vi "Autonomous Independent.vi"() -> ()   [LabVIEW 2013]
doc: "This VI is called when autonomous begins, and will automatically be terminated when autonomous ends. You can carry out timed or sensor driven robot movement independently without needing to return to the caller."
uses:
  <vilib>/Rock Robotics/WPI/SafetyOutput/WPI_SafetyOutputConfigMenu.ctl
  Robot Global Data.vi
  <vilib>/Rock Robotics/WPI/RobotDrive/WPI_RobotDriveGetSetRefNum.vi
  <vilib>/Rock Robotics/WPI/Joystick/WPI_JoystickGetSetRefNum.vi
  <vilib>/Rock Robotics/WPI/RobotDrive/WPI_RobotDriveArcadeDrive_Standard(NoSaturation).vi
panel:
  in  "Mantis_Arm_Move_Position":dbl=69.0
  in  "Max_Position_Error":dbl=5.0 format="%#_13g"
  in  "Shooting_Arm_Position":dbl=95.0
  in  "Min_Wait_Time":dbl=0.75
  in  "Right_Gain":dbl=0.95
  in  "Left_Gain":dbl=1.0
  in  "Backwards":bool
  in  "Invert_Right":bool=TRUE
  in  "Invert_Left":bool=TRUE
  out "Drive_Time_Actual":dbl=4.669
  in  "Loop_Rate":dbl=0.01
  in  "Ramp_Down_Time":dbl=1.0000000000000002
  in  "Hold_Time":dbl=2.85
  in  "Max_Speed":dbl=0.19999999999999968
  in  "Ramp_Up_Time":dbl=0.75
  # "Be sure to right-click and choose Data Operations>>Make Current Value default if you want to save the array values with the VI"
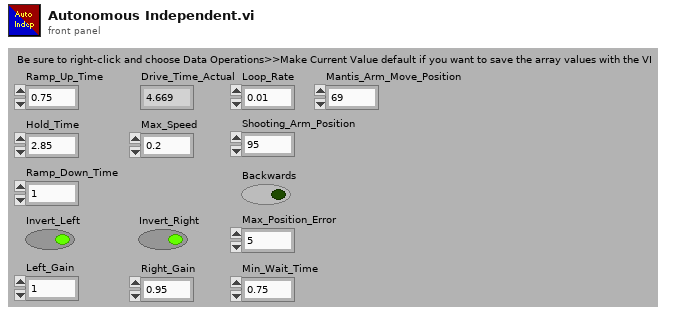
[diagram p1: front panel]
types:
  T1 = typedef "WPI_JoystickDevRef.ctl" = cluster{"Device":T2}
  T2 = typedef "WPI_JoystickDeviceEnum.ctl" = enum16{"USB 1", "USB 2", "USB 3", "USB 4", "Kinect 1", "Kinect 2"}
  T3 = cluster{"axis 1 (x)":dbl, "axis 2 (y)":dbl, "axis 3 (throttle)":dbl, "axis 4":dbl, "axis 5":dbl, "axis 6":dbl}
  T4 = typedef "WPI_RobotDriveDevRef.ctl" = cluster{"DevStatus":errorcluster, "Motors[]":T5[], "Square Inputs":bool, "Max Output":dbl, "Isochronous":bool}
  T5 = typedef "WPI_MotorControlDeviceRef.ctl" = cluster{"DeviceStatus":errorcluster, "Type":enum16{"PWM", "CAN"}, "PWM":cluster{"Digital Module":T6, "PWM Channel":T7, "DeadBand":T8}, "CAN":cluster{"Device Number":u8, "Control Mode":T9, "Semaphore":T10, "Max Vout":dbl}, "Invert":bool, "TransformRef":T11, "InvTransformRef":T11}
  T6 = typedef "FPGA_TypedefDigitalModule.ctl" = enum16{"Digital Module 1", "Digital Module 2"}
  T7 = typedef "FPGA_DIOPWMChannel.ctl" = enum8{"PWM 1", "PWM 2", "PWM 3", "PWM 4", "PWM 5", "PWM 6", "PWM 7", "PWM 8", "PWM 9", "PWM 10", "Invalid"}
  T8 = typedef "WPI_PWMDeadband.ctl" = cluster{"Name":string, "maxPositivePwm":i32, "minPositivePwm":i32, "centerPwm":i32, "maxNegativePwm":i32, "minNegativePwm":i32, "angularRange":u16}
  T9 = typedef "WPI_CANJaguar_ControlMode.ctl" = enum8{"Percent VBus", "Current", "Speed", "Position", "Voltage"}
  T10 = typedef "Semaphore RefNum" = refnum<k1>
  T11 = typedef "WPI_PWMTransform_ConPane.ctl" = refnum<vi>
  T12 = typedef "WPI_SafetyOutputConfigMenu.ctl" = enum16{"Enable", "Disable"}
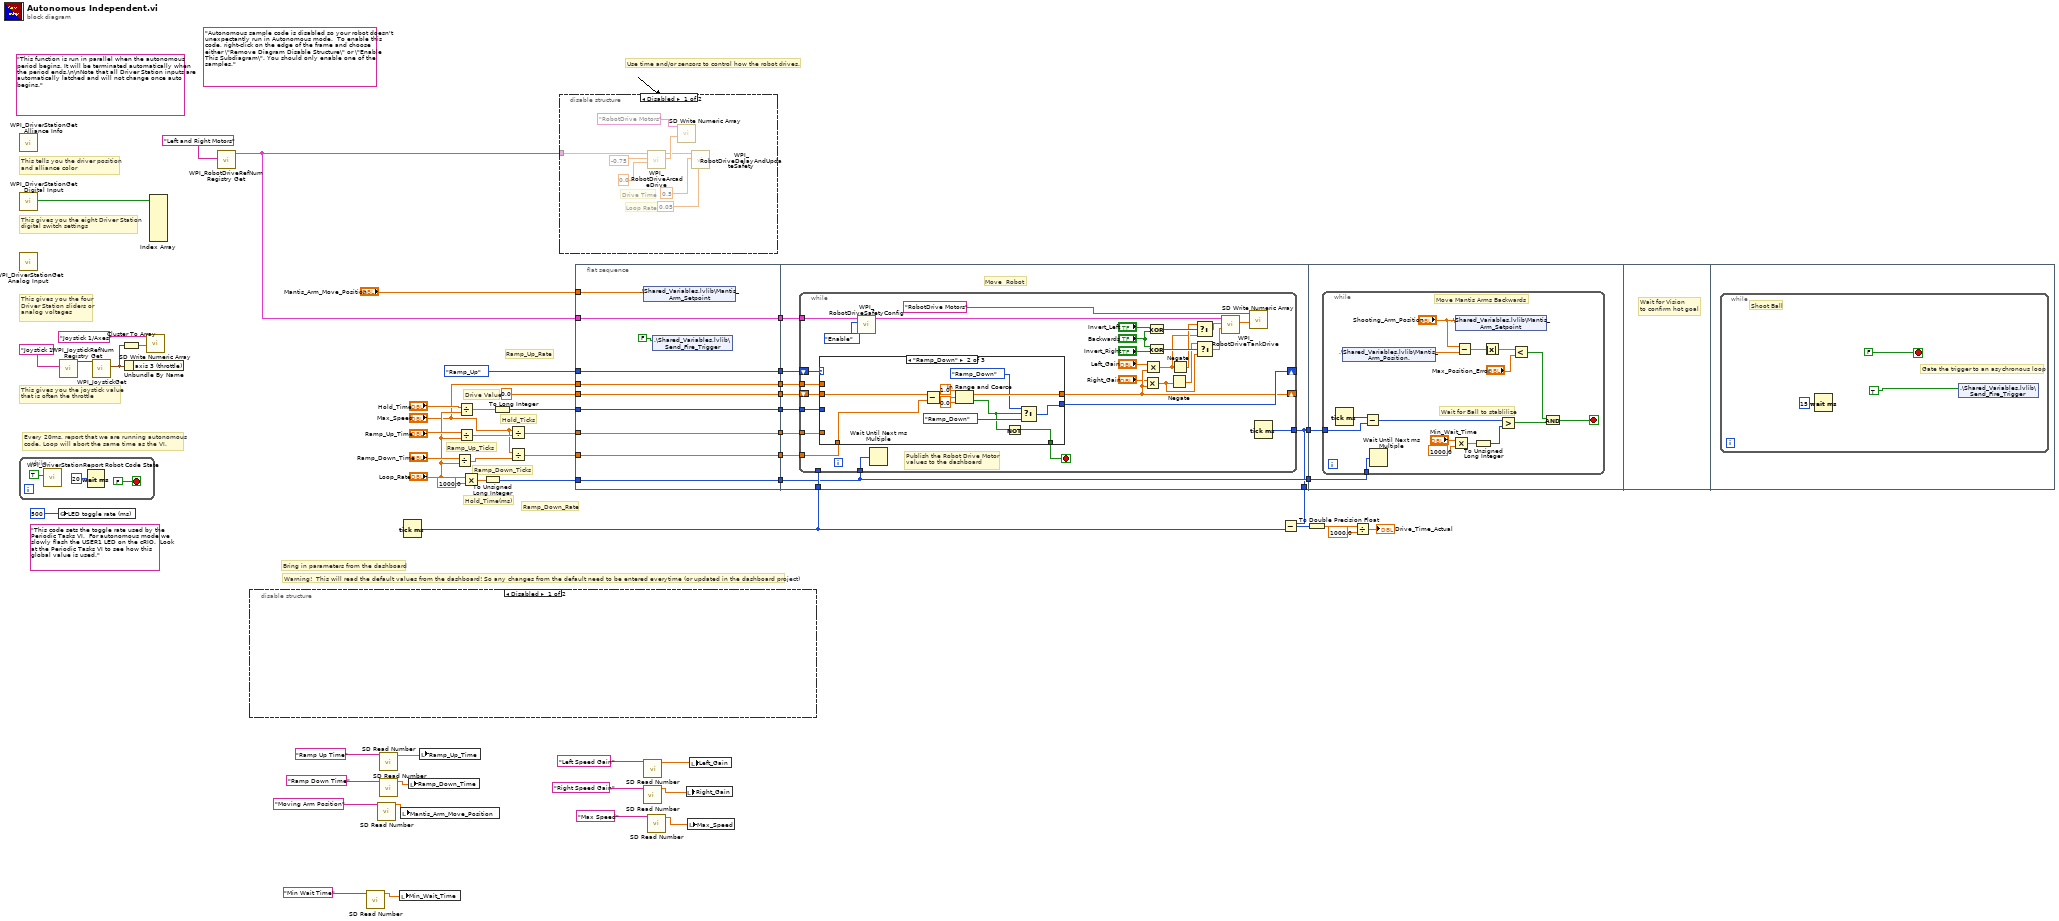
[diagram p0: block diagram]
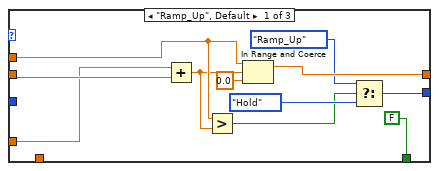
[diagram p3: hidden frame]
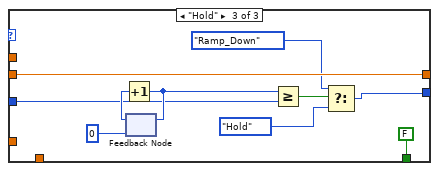
[diagram p4: hidden frame]
diagram:
  (unwired) "This code sets the toggle rate used by the Periodic Tasks VI.  For autonomous mode we slowly flash the USER1 LED on the cRIO.  Look at the Periodic Tasks VI to see how this global value is used."
  (unwired) "Autonomous sample code is disabled so your robot doesn't unexpectantly run in Autonomous mode.  To enable this code, right-click on the edge of the frame and choose either \"Remove Diagram Disable Structure\" or \"Enable This Subdiagram\". You should only enable one of the samples."
  (unwired) "This function is run in parallel when the autonomous period begins. It will be terminated automatically when the period ends.\n\nNote that all Driver Station inputs are automatically latched and will not change once auto begins."
  # "Warning!  This will read the default values from the dashboard! So any changes from the default need to be entered everytime (or updated in the dashboard project)"
  # "Bring in parameters from the dashboard"
  # "Ramp_Up_Rate"
  # "Ramp_Down_Rate"
  # "Ramp_Down_Ticks"
  # "Ramp_Up_Ticks"
  # "Hold_Time(ms)"
  # "Hold_Ticks"
  # "Drive Value"
  # "Every 20ms, report that we are running autonomous\ncode. Loop will abort the same time as the VI."
  # "This gives you the joystick value\nthat is often the throttle"
  # "Use time and/or sensors to control how the robot drives."
  # "This tells you the driver position\nand alliance color"
  # "This gives you the eight Driver Station\ndigital switch settings"
  # "This gives you the four\nDriver Station sliders or\nanalog voltages"
  n1 = while {
    stop <- FALSE stop-if-true
    n2 = call <vilib>:"WPI_DriverStationReport Robot Code State.vi"("Autonomous"=TRUE) -> ()  [unwired: 10 in, 1 out]
    n3 = Wait (ms)(milliseconds to wait=u32 20) -> ()  [unwired: 1 out]
  }
  n4 = call <vilib>:"WPI_DriverStationGet Alliance Info.vi"() -> ()  [unwired: 12 out]
  n5 = call <vilib>:"WPI_DriverStationGet Digital Input.vi"() -> ("Driver Station Digital Input (1-8)"=w56:bool[])  [unwired: 11 out]
  n6 = call <vilib>:"WPI_DriverStationGet Analog Input.vi"() -> ()  [unwired: 12 out]
  n7 = global write "Robot Global Data.vi" "LED toggle rate (ms)"(u32 500 ("LED ms toggle rate")) -> ()
  n8 = call <vilib>:"WPI_JoystickRefNum Registry Get.vi"("refnum name"="Joystick 1") -> ("JoystickDevRef"=w54:T1)  [unwired: 1 in, 9 out]
  n9 = call <vilib>:"WPI_JoystickGet.vi"("JoystickDevRef"=w54) -> ("Axes"=w51:T3)  [unwired: 1 in, 5 out]
  n10 = Cluster To Array(cluster=w51) -> (array=w52:dbl[])
  n11 = Unbundle By Name(w51) -> ()  [unwired: 1 out]
  n12 = call <vilib>:"SD Write Numeric Array.vi"("Numeric Array"=w52, "Name"="Joystick 1/Axes") -> ()  [unwired: 8 in, 2 out]
  n13 = Index Array(array=w56) -> ()  [unwired: 8 in, 8 out]
  n14 = call <vilib>:"WPI_RobotDriveRefNum Registry Get.vi"("refnum name"="Left and Right Motors") -> ("RobotDriveDevRef"=w48:T4)  [unwired: 1 in, 9 out]
  n15 = disable-structure shown="Disabled" {
    frame Disabled {
    }
    frame Enabled {
    }
  }
  n16 = call <vilib>:"SD Read Number.vi"("Name"="Min Wait Time" ("refnum name")) -> ("Numeric"=w8:dbl)  [unwired: 8 in, 2 out]
  n17 = call <vilib>:"SD Read Number.vi"("Name"="Moving Arm Position" ("refnum name")) -> ("Numeric"=w9:dbl)  [unwired: 8 in, 2 out]
  n18 = call <vilib>:"SD Read Number.vi"("Name"="Ramp Up Time" ("refnum name")) -> ("Numeric"=w11:dbl)  [unwired: 8 in, 2 out]
  n19 = call <vilib>:"SD Read Number.vi"("Name"="Ramp Down Time" ("refnum name")) -> ("Numeric"=w10:dbl)  [unwired: 8 in, 2 out]
  n20 = local write "Min_Wait_Time"(w8) -> ()
  n21 = local write "Mantis_Arm_Move_Position"(w9) -> ()
  n22 = Tick Count (ms)() -> (millisecond timer value=w26:u32)
  n23 = local write "Ramp_Down_Time"(w10) -> ()
  n24 = local write "Ramp_Up_Time"(w11) -> ()
  n25 = Divide(x="Ramp_Down_Time", y="Loop_Rate") -> (x/y=w34:dbl)
  n26 = Divide(x="Hold_Time", y="Loop_Rate") -> (x/y=w44:dbl)
  n27 = Divide(x="Ramp_Up_Time", y="Loop_Rate") -> (x/y=w38:dbl)
  n28 = Multiply(x="Loop_Rate", y=1000.0) -> (x*y=w41:dbl)
  n29 = To Unsigned Long Integer(number=w41) -> (unsigned 32bit integer=w40:u32)
  n30 = To Long Integer(number=w44) -> (32bit integer=w43:i32)
  n31 = Divide(x="Max_Speed", y=w38) -> (x/y=w35:dbl)
  n32 = Divide(x="Max_Speed", y=w34) -> (x/y=w32:dbl)
  n33 = disable-structure shown="Disabled" {
    disable-tunnel: w48 -> [w60 _]
    frame Disabled {
      # "Loop Rate"
      # "Drive Time"
      n34 = call-poly <vilib>:"WPI_RobotDriveArcadeDrive.vi"("Y axis value"=0.0 ("X axis value"), "X axis value"=-0.75, "RobotDriveDevRef"=w60) -> ("Motor Values"=w66:dbl[], "RobotDriveDevRef"=w64:T4)  [unwired: 1 in, 6 out]
      n35 = call <vilib>:"SD Write Numeric Array.vi"("Numeric Array"=w66, "Name"="RobotDrive Motors") -> ()  [unwired: 8 in, 2 out]
      n36 = call <vilib>:"WPI_RobotDriveDelayAndUpdateSafety.vi"("Feed time (s)"=0.05, "Delay (s)"=0.5, "RobotDriveDevRef"=w64) -> ()  [unwired: 7 in, 2 out]
    }
    frame Enabled {
    }
  }
  n37 = flat-sequence {
    tunnel: w32 -> [w70]
    tunnel: "Max_Speed" -> [w71]
    tunnel: w35 -> [w72]
    tunnel: w40 -> [w73]
    tunnel: w43 -> [w74]
    tunnel: 0.0 -> [w75]
    tunnel: enum16{"Ramp_Up", "Hold", "Ramp_Down", ""}."Ramp_Up" -> [w76]
    tunnel: w48 -> [w77]
    tunnel: [w77] -> w23
    tunnel: [w76] -> w22
    tunnel: [w75] -> w21
    tunnel: [w74] -> w20
    tunnel: [w73] -> w19
    tunnel: [w72] -> w18
    tunnel: [w71] -> w17
    tunnel: [w70] -> w16
    tunnel: "Mantis_Arm_Move_Position" -> [w69]
    tunnel: [w78] -> w31
    tunnel: w26 -> [w80]
    tunnel: [w79] -> w25
    tunnel: [w78] -> w24
    tunnel: w23 -> [w87]
    tunnel: w22 -> [w86]
    tunnel: w21 -> [w85]
    tunnel: w20 -> [w84]
    tunnel: w19 -> [w79]
    tunnel: w18 -> [w83]
    tunnel: w17 -> [w82]
    tunnel: w16 -> [w81]
    tunnel: w25 -> [w150]
    tunnel: w24 -> [w149]
    frame #0 {
      n38 = shared-variable ".\\Shared_Variables.lvlib\\Mantis_Arm_Setpoint"(w69) -> ()  [unwired: 1 in, 1 out]
      n39 = shared-variable ".\\Shared_Variables.lvlib\\Send_Fire_Trigger"(FALSE ("x")) -> ()  [unwired: 1 in, 1 out]
    }
    frame #1 {
      # "Move  Robot"
      n40 = while {
        tunnel: w87 -> [w114]
        shift-right: [w110] -> _
        shift-left: w86 -> [w112]
        shift-right: [w95] -> _
        shift-left: w85 -> [w111]
        tunnel: w84 -> [w108]
        tunnel: w79 -> [w107]
        tunnel: w83 -> [w106]
        tunnel: w82 -> [w105]
        tunnel: w81 -> [w104]
        tunnel: [w103] -> w78
        tunnel: w80 -> [_]
        stop <- w109 stop-if-true
        # "Publish the Robot Drive Motor\nvalues to the dashboard"
        n41 = case shown="\"Ramp_Down\"" w112 {
          tunnel: w111 -> [w127 w131 w148]
          tunnel: [w125 w136 w148] -> w95
          tunnel: [w124 w135 w142] -> w110
          tunnel: [FALSE w129 FALSE] -> w109
          tunnel: w108 -> [_ _ w139]
          tunnel: w106 -> [w120 _ _]
          tunnel: w105 -> [w119 _ _]
          tunnel: w104 -> [_ w128 _]
          frame "Ramp_Up", Default {
            n42 = Add(x=w120, y=w127) -> (x+y=w118:dbl)
            n43 = Greater?(x=w119, y=w118) -> (0:w117:bool)
            n44 = In Range and Coerce(upper limit=w119, x=w118, lower limit=0.0) -> (coerced(x)=w125:dbl)  [unwired: 1 out]
            n45 = Select(t=enum16{"Ramp_Up", "Hold", "Ramp_Down", ""}."Ramp_Up", s=w117, f=enum16{"Ramp_Up", "Hold", "Ramp_Down", ""}."Hold") -> (s? t:f=w124:enum16{"Ramp_Up", "Hold", "Ramp_Down", ""})
          }
          frame "Ramp_Down" {
            n46 = Subtract(x=w131, y=w128) -> (x-y=w138:dbl)
            n47 = In Range and Coerce(upper limit=1.0, x=w138, lower limit=0.0) -> (coerced(x)=w136:dbl, In Range?=w130:bool)
            n48 = Not(x=w130) -> (.not. x?=w129:bool)
            n49 = Select(t=enum16{"Ramp_Up", "Hold", "Ramp_Down", ""}."Ramp_Down", s=w130, f=enum16{"Ramp_Up", "Hold", "Ramp_Down", ""}."Ramp_Down") -> (s? t:f=w135:enum16{"Ramp_Up", "Hold", "Ramp_Down", ""})
          }
          frame "Hold" {
            n50 = feedback #1(0) -> (w147:i32)
            n51 = Increment(x=w147) -> (x+1=w145:i32)
            n52 = feedback-in #1(w145) -> ()
            n53 = Greater Or Equal?(x=w145, y=w139) -> (x >= y?=w144:bool)
            n54 = Select(t=enum16{"Ramp_Up", "Hold", "Ramp_Down", ""}."Ramp_Down", s=w144, f=enum16{"Ramp_Up", "Hold", "Ramp_Down", ""}."Hold") -> (s? t:f=w142:enum16{"Ramp_Up", "Hold", "Ramp_Down", ""})
          }
        }
        n55 = call <vilib>:"WPI_RobotDriveSafetyConfig.vi"("mode"=WPI_SafetyOutputConfigMenu."Enable", "RobotDriveDevRef"=w114) -> ("RobotDriveDevRef"=w113:T4)  [unwired: 8 in, 1 out]
        n56 = Wait Until Next ms Multiple(millisecond multiple=w107) -> ()  [unwired: 1 out]
        n57 = Multiply(x="Right_Gain", y=w95) -> (x*y=w89:dbl)
        n58 = Multiply(x="Left_Gain", y=w95) -> (x*y=w93:dbl)
        n59 = Exclusive Or(1:"Backwards", 2:"Invert_Left") -> (0:w98:bool)
        n60 = Exclusive Or(1:"Invert_Right", 2:"Backwards") -> (0:w97:bool)
        n61 = Negate(x=w89) -> (-x=w90:dbl)
        n62 = Negate(x=w93) -> (-x=w94:dbl)
        n63 = Select(t=w94, s=w98, f=w93) -> (s? t:f=w101:dbl)
        n64 = Select(t=w90, s=w97, f=w89) -> (s? t:f=w96:dbl)
        n65 = call <vilib>:"WPI_RobotDriveTankDrive.vi"("Right axis value"=w96, "Left axis value"=w101, "RobotDriveDevRef"=w113) -> ("Motor Values"=w115:dbl[])  [unwired: 6 in, 2 out]
        n66 = call <vilib>:"SD Write Numeric Array.vi"("Numeric Array"=w115, "Name"="RobotDrive Motors") -> ()  [unwired: 8 in, 2 out]
        n67 = Tick Count (ms)() -> (millisecond timer value=w103:u32)
      }
    }
    frame #2 {
      n68 = while {
        tunnel: w150 -> [w163]
        tunnel: w149 -> [w161]
        stop <- w157 stop-if-true
        # "Wait for Ball to stablilize"
        # "Move Mantis Arms Backwards"
        n69 = Tick Count (ms)() -> (millisecond timer value=w162:u32)
        n70 = shared-variable ".\\Shared_Variables.lvlib\\Mantis_Arm_Position."() -> (w155:dbl)  [unwired: 1 in, 1 out]
        n71 = Subtract(x=w162, y=w161) -> (x-y=w160:u32)
        n72 = Wait Until Next ms Multiple(millisecond multiple=w163) -> ()  [unwired: 1 out]
        n73 = Multiply(x="Min_Wait_Time", y=1000.0) -> (x*y=w164:dbl)
        n74 = shared-variable ".\\Shared_Variables.lvlib\\Mantis_Arm_Setpoint"("Shooting_Arm_Position") -> ()  [unwired: 1 in, 1 out]
        n75 = Subtract(x="Shooting_Arm_Position", y=w155) -> (x-y=w154:dbl)
        n76 = To Unsigned Long Integer(number=w164) -> (unsigned 32bit integer=w159:u32)
        n77 = Absolute Value(x=w154) -> (abs(x)=w153:dbl)
        n78 = Greater?(x=w160, y=w159) -> (0:w158:bool)
        n79 = Less?(x=w153, y="Max_Position_Error") -> (x < y?=w151:bool)
        n80 = And(x=w151, y=w158) -> (x .and. y?=w157:bool)
      }
    }
    frame #3 {
      # "Wait for Vision\nto confirm hot goal"
    }
    frame #4 {
      n81 = while {
        stop <- FALSE ("x") stop-if-true
        # "Gate the trigger to an asychronous loop"
        # "Shoot Ball"
        n82 = Wait (ms)(milliseconds to wait=u32 15) -> ()  [unwired: 1 out]
        n83 = shared-variable ".\\Shared_Variables.lvlib\\Send_Fire_Trigger"(TRUE ("x")) -> ()  [unwired: 1 in, 1 out]
      }
    }
  }
  n84 = call <vilib>:"SD Read Number.vi"("Name"="Right Speed Gain" ("refnum name")) -> ("Numeric"=w3:dbl)  [unwired: 8 in, 2 out]
  n85 = call <vilib>:"SD Read Number.vi"("Name"="Left Speed Gain" ("refnum name")) -> ("Numeric"=w4:dbl)  [unwired: 8 in, 2 out]
  n86 = call <vilib>:"SD Read Number.vi"("Name"="Max Speed" ("refnum name")) -> ("Numeric"=w1:dbl)  [unwired: 8 in, 2 out]
  n87 = local write "Right_Gain"(w3) -> ()
  n88 = local write "Max_Speed"(w1) -> ()
  n89 = local write "Left_Gain"(w4) -> ()
  n90 = Subtract(x=w31, y=w26) -> (x-y=w30:u32)
  n91 = To Double Precision Float(number=w30) -> (double precision float=w29:dbl)
  n92 = Divide(x=w29, y=1000.0) -> (x/y=→"Drive_Time_Actual":dbl)
